vi "FTW-Actor-AddJob-Next.vi"(1 "Add Next in Job Queue":string, 3 "FTW Actor":refnum<class "FTW-Actor.lvclass">) -> (0 "FTW Actor out":refnum<class "FTW-Actor.lvclass">)   [LabVIEW 2015, in "FTW-Actor.lvclass"]
uses:
  FTW-Actor.lvclass
  FTW-Actor.lvclass/FTW-Actor.ctl
  Sequencer/FTW-Sequencer.lvclass/FTW-Sequencer.ctl
  Sequencer/FTW-Sequencer.lvclass
panel:
  # "Inputs"
  # "Outputs"
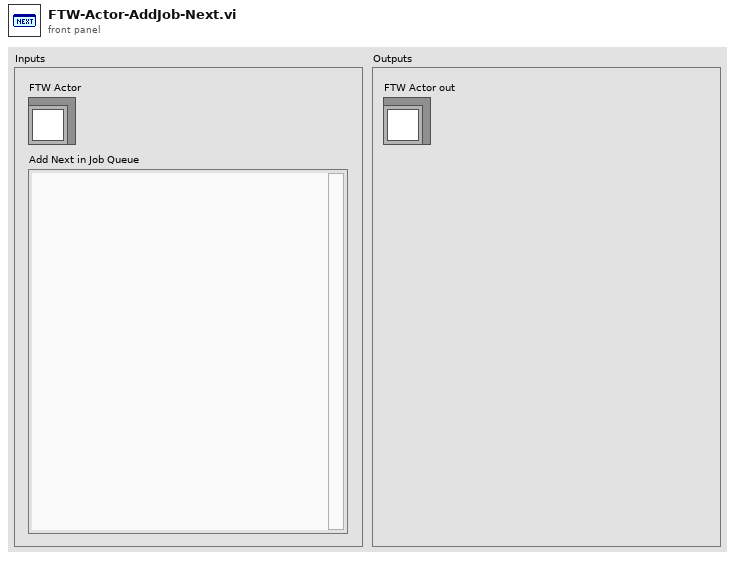
[diagram p1: front panel]
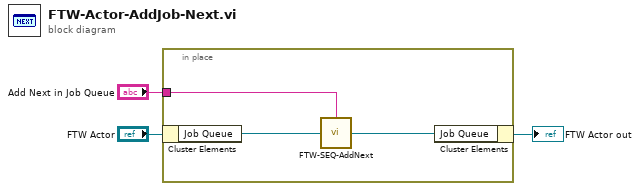
[diagram p0: block diagram]
diagram:
  n1 = in-place {
    in-place-border: "Add Next in Job Queue" -> [w4]
    n2 = in-place-cluster #1("FTW Actor") -> ("Job Queue"=w6:refnum<class "FTW-Sequencer.lvclass">)
    n3 = call "FTW-SEQ-AddNext.vi"("Add Next in Sequence"=w4, "Sequencer"=w6) -> ("Sequencer out"=w5:refnum<class "FTW-Sequencer.lvclass">)  [unwired: 2 in]
    n4 = in-place-cluster #1("Job Queue"=w5) -> (→"FTW Actor out":refnum<class "FTW-Actor.lvclass">)
  }
